vi "AnalyseRamp.vi"() -> ()   [LabVIEW 2024]
uses:
  controls/TestCycleParams.ctl
  controls/SurviveCycleParams.ctl
  controls/ControlInput.ctl
  <vilib>/Waveform/WDTOps.llb/WDT Index Channel DBL.vi
  <vilib>/measure/mascope.llb/Transition Measurements 1 chan.vi
  <vilib>/Waveform/WDTOps.llb/WDT Get Waveform Subset DBL.vi
  <vilib>/measure/NI_MAPro.lvlib
panel:
  out "Test Ramp(deg/min)":dbl=0.8041305762794494
  out "Hot Overshoot":dbl=4.046999999999997
  out "Heating (deg/min)":dbl=2.4799315816035765
  out "Cold Overshoot":dbl=-4.6510000000000105
  out "Cooling (deg/min)":dbl=3.7458769486300576
  in  "Tab Control":enum32{"All", "Control", "Control 2"}(tab)=enum."Control"
  out "All Signals":dynamicdata(graph)=[{"t0"=timestamp(3817282106.814144 s since 1904-01-01), "dt"=5.0, "Y"=array[18039 elements], "attributes"=variant("NI_ChannelName"=variant(string " 3A"), "NI_ExpIsRelativeTime"=variant(bool FALSE), "NI_ExpStartTimeStamp"=variant(timestamp timestamp(3817282106.814144 s since 1904-01-01)), "NI_ExpTimeStamp"=variant(timestamp timestamp(3817282106.814144 s since 1904-01-01)), "NI_ExpXDimension"=variant(string "t"))}, {"t0"=timestamp(3817282106.814144 s since 1904-01-01), "dt"=5.0, "Y"=array[18039 elements], "attributes"=variant("NI_ChannelName"=variant(string " 3B"), "NI_ExpIsRelativeTime"=variant(bool FALSE), "NI_ExpStartTimeStamp"=variant(timestamp timestamp(3817282106.814144 s since 1904-01-01)), "NI_ExpTimeStamp"=variant(timestamp timestamp(3817282106.814144 s since 1904-01-01)), "NI_ExpXDimension"=variant(string "t"))}, {"t0"=timestamp(3817282106.814144 s since 1904-01-01), "dt"=5.0, "Y"=array[18039 elements], "attributes"=variant("NI_ChannelName"=variant(string " 3C"), "NI_ExpIsRelativeTime"=variant(bool FALSE), "NI_ExpStartTimeStamp"=variant(timestamp timestamp(3817282106.814144 s since 1904-01-01)), "NI_ExpTimeStamp"=variant(timestamp timestamp(3817282106.814144 s since 1904-01-01)), "NI_ExpXDimension"=variant(string "t"))}, {"t0"=timestamp(3817282106.814144 s since 1904-01-01), "dt"=5.0, "Y"=array[18039 elements], "attributes"=variant("NI_ChannelName"=variant(string " 3D"), "NI_ExpIsRelativeTime"=variant(bool FALSE), "NI_ExpStartTimeStamp"=variant(timestamp timestamp(3817282106.814144 s since 1904-01-01)), "NI_ExpTimeStamp"=variant(timestamp timestamp(3817282106.814144 s since 1904-01-01)), "NI_ExpXDimension"=variant(string "t"))}, {"t0"=timestamp(3817282106.814144 s since 1904-01-01), "dt"=5.0, "Y"=array[18039 elements], "attributes"=variant("NI_ChannelName"=variant(string " 4A"), "NI_ExpIsRelativeTime"=variant(bool FALSE), "NI_ExpStartTimeStamp"=variant(timestamp timestamp(3817282106.814144 s since 1904-01-01)), "NI_ExpTimeStamp"=variant(timestamp timestamp(3817282106.814144 s since 1904-01-01)), "NI_ExpXDimension"=variant(string "t"))}, {"t0"=timestamp(3817282106.814144 s since 1904-01-01), "dt"=5.0, "Y"=array[18039 elements], "attributes"=variant("NI_ChannelName"=variant(string " 4B"), "NI_ExpIsRelativeTime"=variant(bool FALSE), "NI_ExpStartTimeStamp"=variant(timestamp timestamp(3817282106.814144 s since 1904-01-01)), "NI_ExpTimeStamp"=variant(timestamp timestamp(3817282106.814144 s since 1904-01-01)), "NI_ExpXDimension"=variant(string "t"))}, {"t0"=timestamp(3817282106.814144 s since 1904-01-01), "dt"=5.0, "Y"=array[18039 elements], "attributes"=variant("NI_ChannelName"=variant(string " 4C"), "NI_ExpIsRelativeTime"=variant(bool FALSE), "NI_ExpStartTimeStamp"=variant(timestamp timestamp(3817282106.814144 s since 1904-01-01)), "NI_ExpTimeStamp"=variant(timestamp timestamp(3817282106.814144 s since 1904-01-01)), "NI_ExpXDimension"=variant(string "t"))}, {"t0"=timestamp(3817282106.814144 s since 1904-01-01), "dt"=5.0, "Y"=array[18039 elements], "attributes"=variant("NI_ChannelName"=variant(string " 4D"), "NI_ExpIsRelativeTime"=variant(bool FALSE), "NI_ExpStartTimeStamp"=variant(timestamp timestamp(3817282106.814144 s since 1904-01-01)), "NI_ExpTimeStamp"=variant(timestamp timestamp(3817282106.814144 s since 1904-01-01)), "NI_ExpXDimension"=variant(string "t"))}, {"t0"=timestamp(3817282106.552352 s since 1904-01-01), "dt"=5.0, "Y"=array[18039 elements], "attributes"=variant("NI_ChannelName"=variant(string "Backing Pressure"), "NI_ExpIsRelativeTime"=variant(bool FALSE), "NI_ExpStartTimeStamp"=variant(timestamp timestamp(3817282106.552352 s since 1904-01-01)), "NI_ExpTimeStamp"=variant(timestamp timestamp(3817282106.552352 s since 1904-01-01)), "NI_ExpXDimension"=variant(string "t"))}, {"t0"=timestamp(3817282106.552352 s since 1904-01-01), "dt"=5.0, "Y"=array[18039 elements], "attributes"=variant("NI_ChannelName"=variant(string "Chamber Pressure"), "NI_ExpIsRelativeTime"=variant(bool FALSE), "NI_ExpStartTimeStamp"=variant(timestamp timestamp(3817282106.552352 s since 1904-01-01)), "NI_ExpTimeStamp"=variant(timestamp timestamp(3817282106.552352 s since 1904-01-01)), "NI_ExpXDimension"=variant(string "t"))}, {"t0"=timestamp(3817282106.814144 s since 1904-01-01), "dt"=5.0, "Y"=array[18039 elements], "attributes"=variant("NI_ChannelName"=variant(string "Relays"), "NI_ExpIsRelativeTime"=variant(bool FALSE), "NI_ExpStartTimeStamp"=variant(timestamp timestamp(3817282106.814144 s since 1904-01-01)), "NI_ExpTimeStamp"=variant(timestamp timestamp(3817282106.814144 s since 1904-01-01)), "NI_ExpXDimension"=variant(string "t"))}]
  out "ControlChannel":waveform(dbl)(graph)={"t0"=timestamp(3817282106.814144 s since 1904-01-01), "dt"=5.0, "Y"=array[18039 elements], "attributes"=variant("NI_ChannelName"=variant(string " 3C"), "NI_ExpIsRelativeTime"=variant(bool FALSE), "NI_ExpStartTimeStamp"=variant(timestamp timestamp(3817282106.814144 s since 1904-01-01)), "NI_ExpTimeStamp"=variant(timestamp timestamp(3817282106.814144 s since 1904-01-01)), "NI_ExpXDimension"=variant(string "t"))}
  in  "TestCycleParameters":T1={"TAmb"=20.0, "HeaterTestTemp"=-80.0, "HeaterTestDwell"=30, "HeaterTestDuration"=15, "MinOpTemp"=-50.0, "MinOpDwell(min)"=30, "TestHeatingRate (deg/min)"=0.8, "SurviveCycleParameters"={"MinSurviveTemp"=-131.5, "MinSurvive Dwell"=10, "MaxOpTemp"=25.0, "MaxOpDwell"=30, "ControlInput"=2, "ColdStandOff"=4.0, "HotStandoff"=5.0, "SteadyPWM"=20, "MaxCoolingRate (deg/min)"=3.75, "MaxHeatingRate (deg/min)"=2.5}} {"SurviveCycleParameters"."SteadyPWM" min=0 max=100 step=1; "SurviveCycleParameters"."ControlInput" items=["3A", "3B", "3C", "3D", "4A", "4B", "4C", "4D"]}
  in  "ControlChannel":u16(ring)=2 items=[" 3A", " 3B", " 3C", " 3D", " 4A", " 4B", " 4C", " 4D", "Backing Pressure", "Chamber Pressure", "Relays"]
  in  "Path":path=path "C:/Users/dpl/OneDrive - Aberystwyth University/Documents/LabVIEW Data/ThermalVacSystem/testCycleLoop2.tdms"
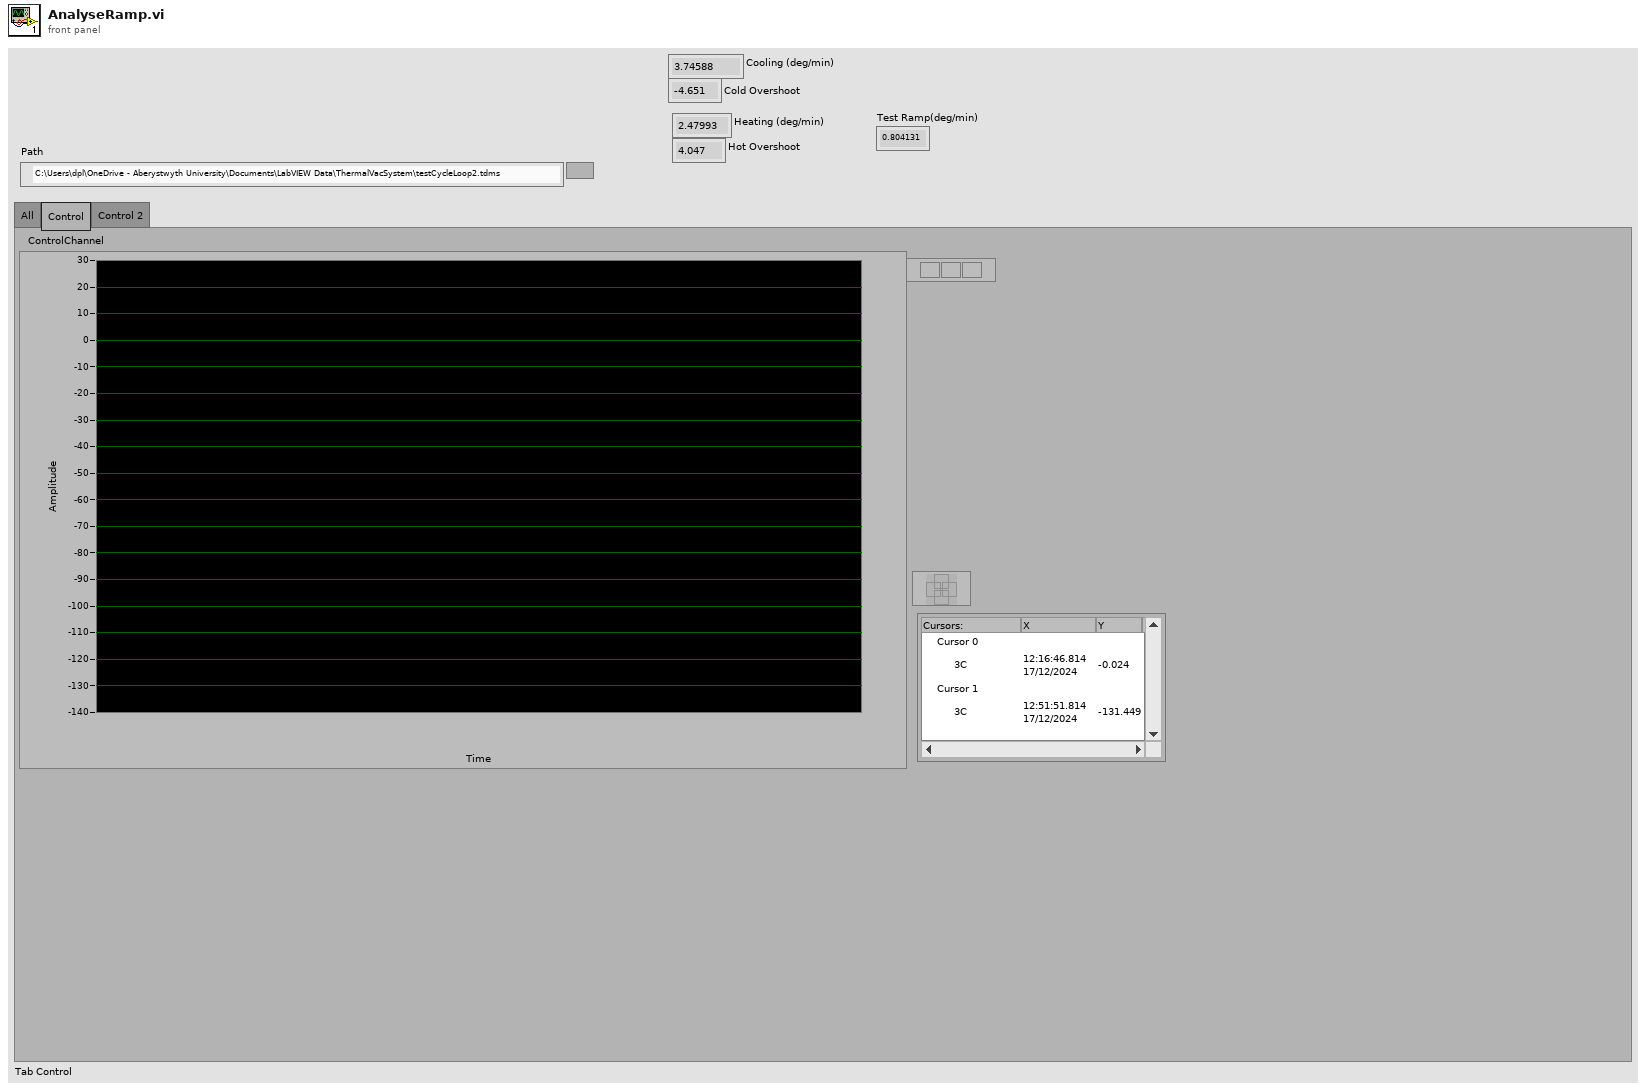
[diagram p1: front panel]
types:
  T1 = typedef "TestCycleParams.ctl" = cluster{"TAmb":dbl, "HeaterTestTemp":dbl, "HeaterTestDwell":i32, "HeaterTestDuration":i32, "MinOpTemp":dbl, "MinOpDwell(min)":i32, "TestHeatingRate (deg/min)":dbl, "SurviveCycleParameters":T2}
  T2 = typedef "SurviveCycleParams.ctl" = cluster{"MinSurviveTemp":dbl, "MinSurvive Dwell":i32, "MaxOpTemp":dbl, "MaxOpDwell":i32, "ControlInput":T3, "ColdStandOff":dbl, "HotStandoff":dbl, "SteadyPWM":i32, "MaxCoolingRate (deg/min)":dbl, "MaxHeatingRate (deg/min)":dbl}
  T3 = typedef "ControlInput.ctl" = u16
  T4 = cluster{"high ref level":dbl, "mid ref level":dbl, "low ref level":dbl, "ref units":u16}
  T5 = cluster{"start time":dbl, "end time":dbl, "ref levels":cluster{"high ref level":dbl, "mid ref level":dbl, "low ref level":dbl, "ref units":u16}}
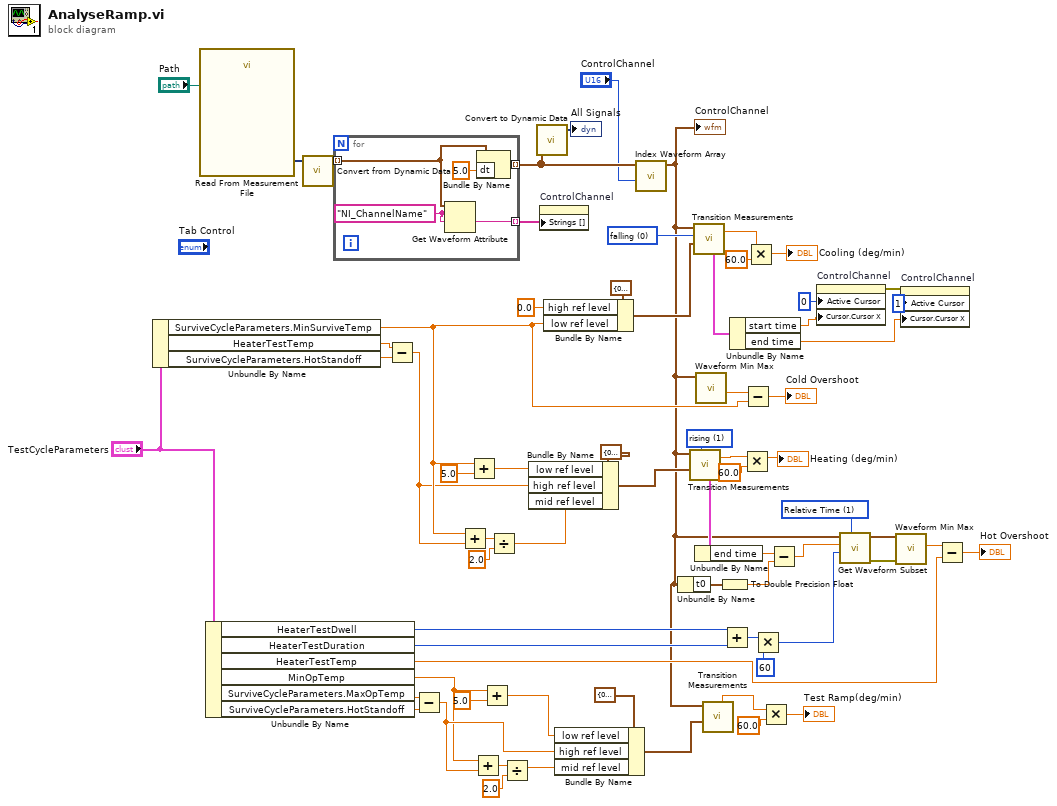
[diagram p0: block diagram]
diagram:
  w32 = u16 1 items=["Samples", "Relative Time"] ("start/duration format")
  w47 = u16 1 items=["falling", "rising"] ("polarity (rising)")
  w64 = u16 0 items=["falling", "rising"] ("polarity (rising)")
  n1 = Unbundle By Name("TestCycleParameters") -> ("SurviveCycleParameters.MinSurviveTemp"=w39:dbl, "HeaterTestTemp"=w34:dbl, "SurviveCycleParameters.HotStandoff"=w33:dbl)
  n2 = call "Read From Measurement File"("Filename"="Path") -> ("Signals"=w68:dynamicdata)  [unwired: 5 in, 5 out]
  n3 = Unbundle By Name("TestCycleParameters") -> ("HeaterTestDwell"=w25:i32, "HeaterTestDuration"=w24:i32, "HeaterTestTemp"=w17:dbl, "MinOpTemp"=w4:dbl, "SurviveCycleParameters.MaxOpTemp"=w8:dbl, "SurviveCycleParameters.HotStandoff"=w9:dbl)
  n4 = call "Convert from Dynamic Data"("Dynamic Data Type"=w68) -> ("Array of Waveform"=w67:waveform(dbl)[])  [unwired: 3 in]
  n5 = for {
    tunnel: w67 -> [w72] mode=indexing
    tunnel: [w73] -> w50 mode=indexing
    tunnel: [w70] -> w66 mode=indexing
    w71 = "NI_ChannelName" ("name")
    n6 = Get Waveform Attribute(5:w71, 6:w71, 7:w72) -> (1:w70:string)  [unwired: 1 in, 3 out]
    n7 = Bundle By Name(cluster=w72, "dt"=5.0) -> (w73:waveform(dbl))
  }
  n8 = Subtract(x=w34, y=w33) -> (x-y=w35:dbl)
  n9 = Subtract(x=w8, y=w9) -> (x-y=w6:dbl)
  n10 = Add(x=w39, y=w35) -> (x+y=w38:dbl)
  n11 = Add(x=w39, y=5.0) -> (x+y=w45:dbl)
  n12 = Add(x=w4, y=w6) -> (x+y=w13:dbl)
  n13 = Add(x=w4, y=5.0) -> (x+y=w7:dbl)
  n14 = Divide(x=w38, y=2.0) -> (x/y=w36:dbl)
  n15 = Divide(x=w13, y=2.0) -> (x/y=w5:dbl)
  n16 = Bundle By Name(cluster=T4 {"high ref level"=0.0, "mid ref level"=0.0, "low ref level"=-120.0, "ref units"=0} ("reference levels"), "low ref level"=w45, "high ref level"=w35, "mid ref level"=w36) -> (w43:T4)
  n17 = call "Convert to Dynamic Data"("Array of Waveforms"=w50) -> ("Dynamic Data Type"=→"All Signals":dynamicdata)  [unwired: 3 in]
  n18 = property on="ControlChannel" class="Ring (strict)"("Strings []"=w66) -> ()  [unwired: 2 in, 2 out]
  n19 = Bundle By Name(cluster=T4 {"high ref level"=0.0, "mid ref level"=0.0, "low ref level"=-120.0, "ref units"=0} ("reference levels"), "high ref level"=0.0, "low ref level"=w39) -> (w59:T4)
  n20 = Bundle By Name(cluster=T4 {"high ref level"=0.0, "mid ref level"=0.0, "low ref level"=-120.0, "ref units"=0} ("reference levels"), "low ref level"=w7, "high ref level"=w6, "mid ref level"=w5) -> (w10:T4)
  n21 = call-poly <vilib>:"Index Waveform Array.vi"("index"="ControlChannel", "waveform array"=w50) -> ("waveform"=w15:waveform(dbl))  [unwired: 8 in, 1 out]
  "ControlChannel" <- w15
  n22 = Unbundle By Name(w15) -> ("t0"=w29:timestamp)
  n23 = call-poly <vilib>:"Transition Measurements.vi"("reference levels"=w43, "polarity (rising)"=w47, "signal in"=w15) -> ("measurement info"=w31:T5, "slope"=w42:dbl)  [unwired: 3 in, 4 out]
  n24 = call-poly <vilib>:"Transition Measurements.vi"("reference levels"=w59, "polarity (rising)"=w64, "signal in"=w15) -> ("measurement info"=w62:T5, "slope"=w63:dbl)  [unwired: 3 in, 4 out]
  n25 = Unbundle By Name(w31) -> ("end time"=w30:dbl)
  n26 = call <vilib>:"Waveform Min Max.vi"("waveform in"=w15) -> ("Y min"=w52:dbl)  [unwired: 5 in, 5 out]
  n27 = call-poly <vilib>:"Transition Measurements.vi"("reference levels"=w10, "signal in"=w15) -> ("slope"=w2:dbl)  [unwired: 4 in, 5 out]
  n28 = To Double Precision Float(number=w29) -> (double precision float=w28:dbl)
  n29 = Add(x=w25, y=w24) -> (x+y=w23:i32)
  n30 = Unbundle By Name(w62) -> ("start time"=w56:dbl, "end time"=w48:dbl)
  n31 = Multiply(x=w42, y=60.0) -> (x*y=→"Heating (deg/min)":dbl)
  n32 = Subtract(x=w52, y=w39) -> (x-y=→"Cold Overshoot":dbl)
  n33 = Multiply(x=w63, y=60.0) -> (x*y=→"Cooling (deg/min)":dbl)
  n34 = Multiply(x=w23, y=60) -> (x*y=w21:i32)
  n35 = Multiply(x=w2, y=60.0) -> (x*y=→"Test Ramp(deg/min)":dbl)
  n36 = Subtract(x=w30, y=w28) -> (x-y=w27:dbl)
  n37 = property on="ControlChannel" class="WFGraph (strict)"("Active Cursor"=u32 0, "Cursor.Cursor X"=w56) -> (error out=w57:errorcluster)  [unwired: 2 in, 1 out]
  n38 = call-poly <vilib>:"Get Waveform Subset.vi"("start/duration format"=w32, "duration"=w21, "start samples/time"=w27, "waveform in"=w15) -> ("error out"=w20:errorcluster, "waveform out"=w19:waveform(dbl))  [unwired: 2 in, 2 out]
  n39 = call <vilib>:"Waveform Min Max.vi"("error in (no error)"=w20, "waveform in"=w19) -> ("Y max"=w18:dbl)  [unwired: 4 in, 5 out]
  n40 = property on="ControlChannel" class="WFGraph (strict)"(error in=w57, "Active Cursor"=u32 1, "Cursor.Cursor X"=w48) -> ()  [unwired: 1 in, 2 out]
  n41 = Subtract(x=w18, y=w17) -> (x-y=→"Hot Overshoot":dbl)
